vi "TEMOCR-Process One Signal.vi"(0 "State In":T1, 5 "array":dbl[](array[numeric]), 7 "index":i32, 9 "length":i32, 11 "Fs (Hz)":dbl, 12 "Analysis":T2) -> (4 "+Freq. Mag of FFT (dB rms)":dbl[](array[numeric]) format="%.2f", 10 "Freq (Hz)":dbl[](array[numeric]))   [LabVIEW 2015]
uses:
  Typedefs/TEMOCR-Analysis.ctl
  Typedefs/TEMOCR-Analysis State.ctl
  <vilib>/Analysis/3filter.llb/Filter Passband Type.ctl
  <vilib>/Analysis/baseanly.llb/Mean (DBL).vi
  <vilib>/Analysis/4window.llb/Hanning Window (DBL).vi
  <vilib>/Analysis/4window.llb/Hamming Window (DBL).vi
  <vilib>/Analysis/4window.llb/AllCosWindow (DBL).vi
  <vilib>/Analysis/3filter.llb/Butterworth Filter (DBL).vi
  Utility VIs/Math VIs/FFT x(t) to dB,Degrees (1D).vi
  Utility VIs/Math VIs/interp1 (1D).vi
  <vilib>/Analysis/NI_AALPro.lvlib
  <vilib>/Analysis/NI_AALBase.lvlib
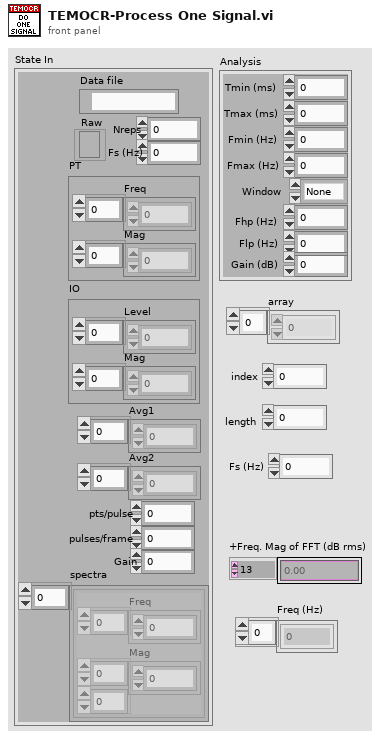
[diagram p1: front panel]
types:
  T1 = typedef "TEMOCR-Analysis State.ctl" = cluster{"Data file":path, "Raw":refnum<file>, "PT":cluster{"Freq":dbl[], "Mag":dbl[]}, "IO":cluster{"Level":dbl[], "Mag":dbl[]}, "Nreps":i32, "Fs (Hz)":dbl, "Avg1":dbl[], "pts/pulse":i32, "pulses/frame":i32, "Avg2":dbl[], "Gain":dbl, "spectra":cluster{"Freq":dbl[], "Mag":dbl[][]}[]}
  T2 = typedef "TEMOCR-Analysis.ctl" = cluster{"Tmin (ms)":dbl, "Tmax (ms)":dbl, "Fmin (Hz)":dbl, "Fmax (Hz)":dbl, "Window":enum16{"None", "Hanning", "Hamming"}, "Fhp (Hz)":dbl, "Flp (Hz)":dbl, "Gain (dB)":dbl}
  T3 = typedef "NI_AALBase.lvlib/Filter Passband Type.ctl" = enum32{"Lowpass", "Highpass", "Bandpass", "Bandstop"}
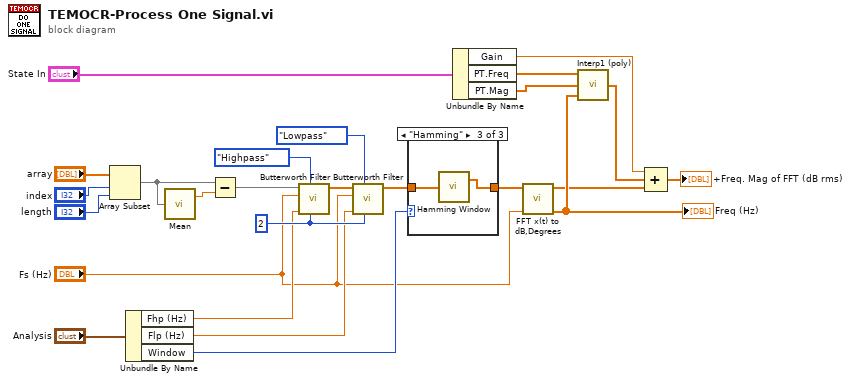
[diagram p0: block diagram]
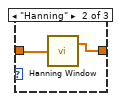
[diagram p3: hidden frame]
diagram:
  w20 = 2 ("order")
  n1 = Array Subset(array="array", index="index", length="length") -> (w9:dbl[])
  n2 = Unbundle By Name("Analysis") -> ("Fhp (Hz)"=w18:dbl, "Flp (Hz)"=w17:dbl, "Window"=w25:enum16{"None", "Hanning", "Hamming"})
  n3 = call-poly <vilib>:"Mean.vi"("X"=w9) -> ("mean"=w10:dbl)  [unwired: 1 out]
  n4 = Subtract(x=w9, y=w10) -> (x-y=w11:dbl[])
  n5 = call-poly <vilib>:"Butterworth Filter.vi"("order"=w20, "filter type"=Filter_Passband_Type."Highpass", "low cutoff freq: fl"=w18, "sampling freq: fs"="Fs (Hz)", "X"=w11) -> ("Filtered X"=w22:dbl[])  [unwired: 3 in, 1 out]
  n6 = call-poly <vilib>:"Butterworth Filter.vi"("order"=w20, "filter type"=Filter_Passband_Type."Lowpass", "low cutoff freq: fl"=w17, "sampling freq: fs"="Fs (Hz)", "X"=w22) -> ("Filtered X"=w21:dbl[])  [unwired: 3 in, 1 out]
  n7 = case shown="\"Hamming\"" w25 {
    tunnel: w21 -> [w26 w28 w30]
    tunnel: [w26 w27 w29] -> w24
    frame "None", Default {
    }
    frame "Hanning" {
      n8 = call-poly <vilib>:"Hanning Window.vi"("X"=w28) -> ("Windowed X"=w27:dbl[])  [unwired: 1 out]
    }
    frame "Hamming" {
      n9 = call-poly <vilib>:"Hamming Window.vi"("X"=w30) -> ("Windowed X"=w29:dbl[])  [unwired: 1 out]
    }
  }
  n10 = Unbundle By Name("State In") -> ("Gain"=w1:dbl, "PT.Freq"=w8:dbl[], "PT.Mag"=w7:dbl[])
  n11 = call-poly "FFT x(t) to dB,Degrees.vi"("Fs (Hz)"="Fs (Hz)", "X"=w24) -> ("Freq (Hz)"=w5:dbl[], "+Freq. Mag of FFT (dB rms)"=w4:dbl[])  [unwired: 7 in, 1 out]
  "Freq (Hz)" <- w5
  n12 = call-poly "Interp1 (poly).vi"("X"=w8, "Y"=w7, "U"=w5) -> ("V"=w2:dbl[])  [unwired: 2 in]
  n13 = Compound Arithmetic op=ADD(w1, w2, w4) -> (→"+Freq. Mag of FFT (dB rms)":dbl[])
